vi "StateMachine_v01.vi"() -> ()   [LabVIEW 2014]
uses:
  StateMachine1Control.ctl
panel:
  out "ensaio":bool
  in  "waiting time":u32
  in  "currentCycleCtr":u32
  out "freio":bool
  in  "velocidade 2":u32
  out "velocidade":u32
  out "motor":bool
  in  "velocidade_inferior":u32
  in  "velocidade_superior":u32
  out "totalCycle":string
  out "currentCycle":string
  in  "numberOfCycles":u32 max=999 step=1 format="%0d"
  in  "stopButton":bool
  in  "startButton":bool
  out "state":T1
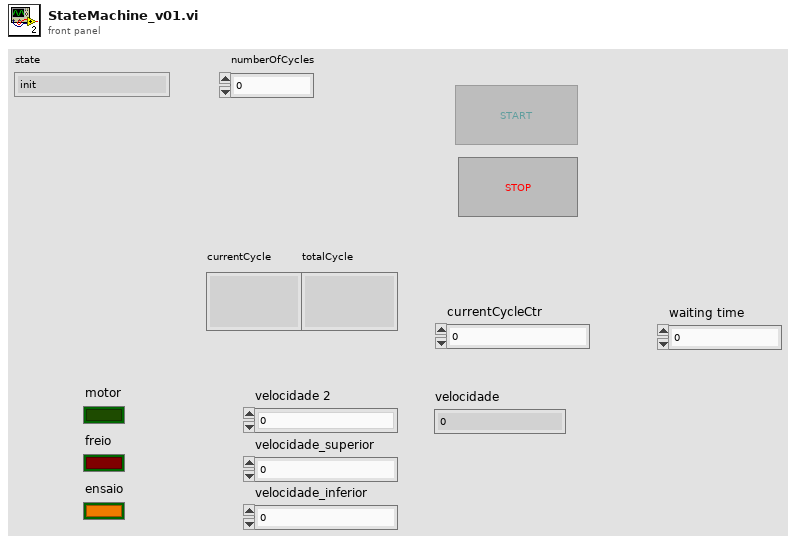
[diagram p1: front panel]
types:
  T1 = typedef "StateMachine1Control.ctl" = enum16{"init", "ready", "start motor cycle", "acquiring data", "start brake cycle", "finish", "shutdown"}
  T2 = enum8{"Enabled", "Disabled", "Disabled and Grayed Out"}
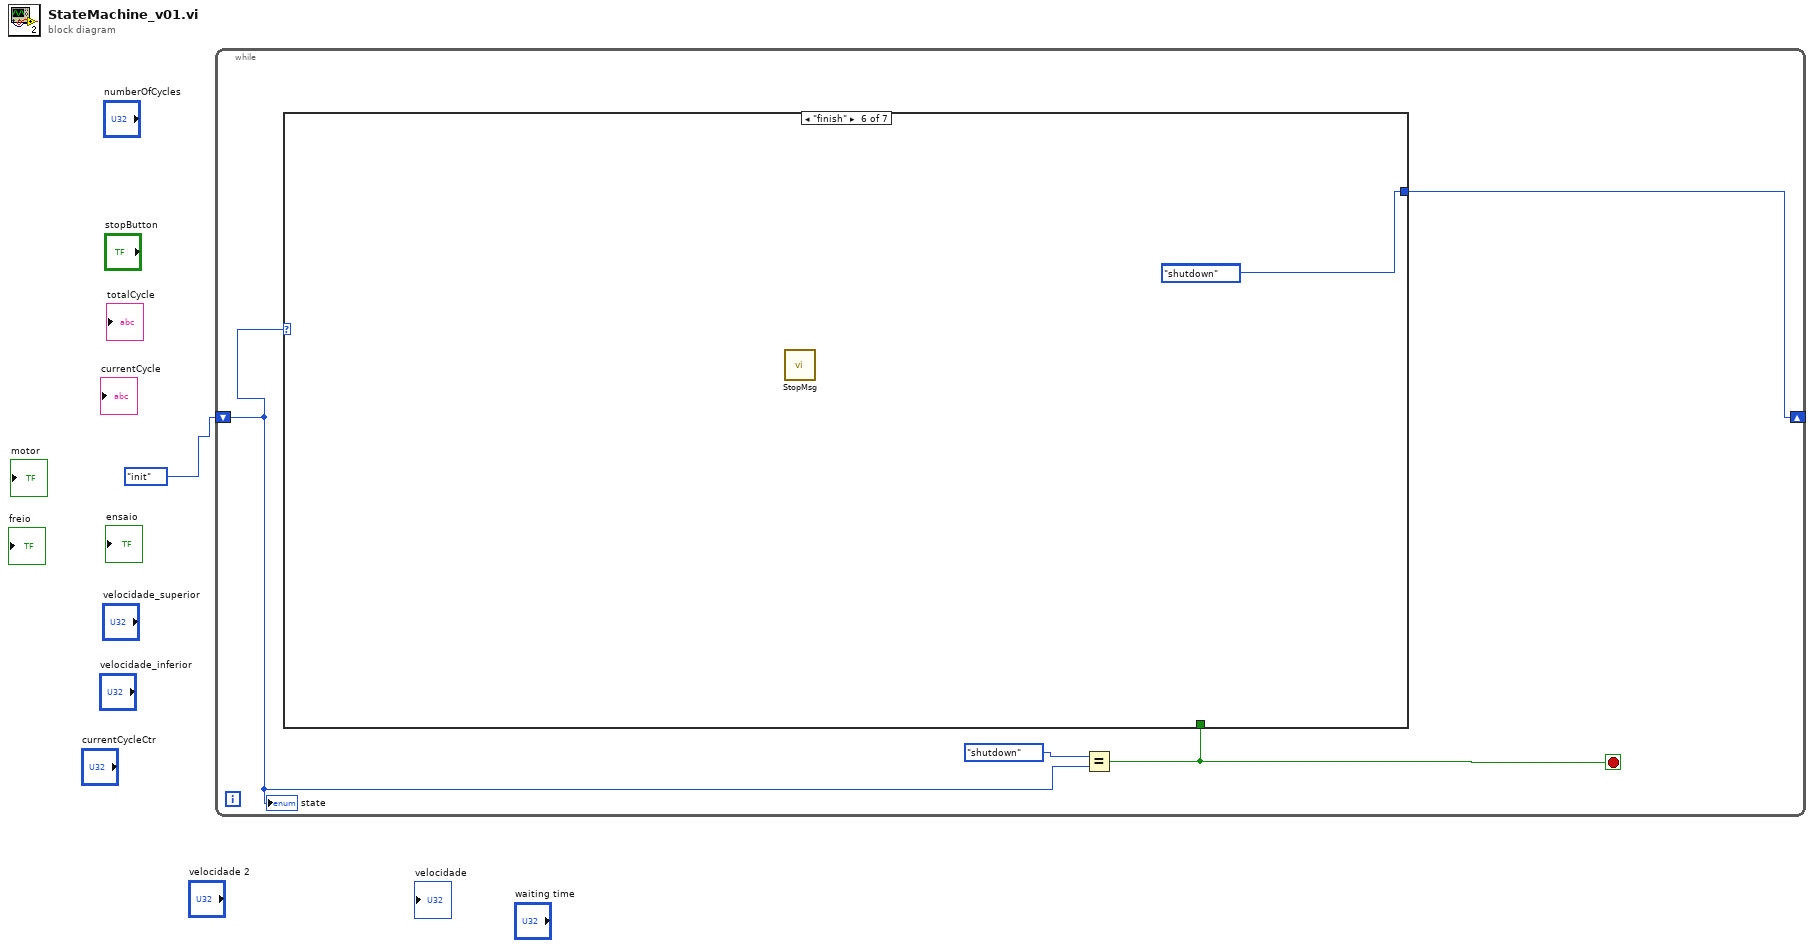
[diagram p0: block diagram]
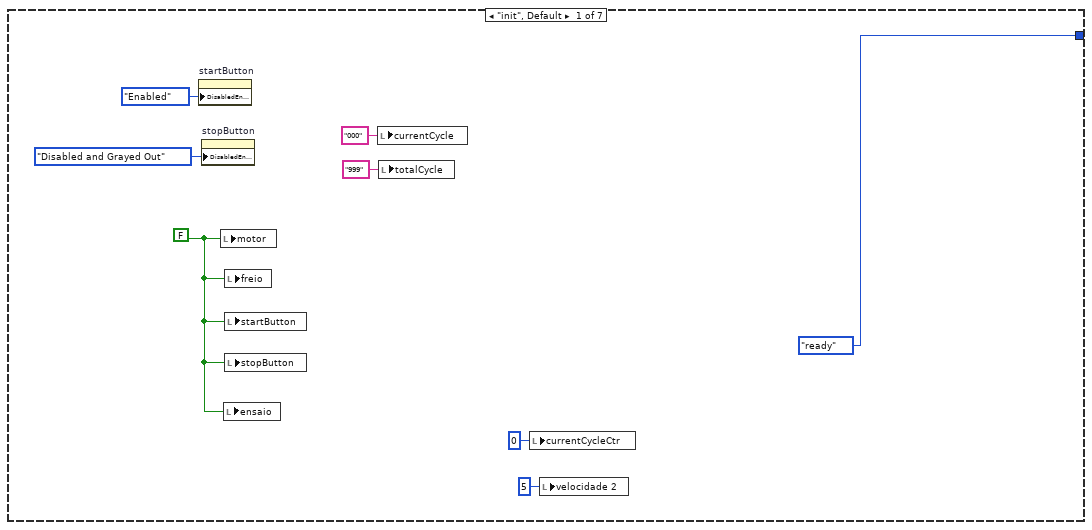
[diagram p2: hidden frame]
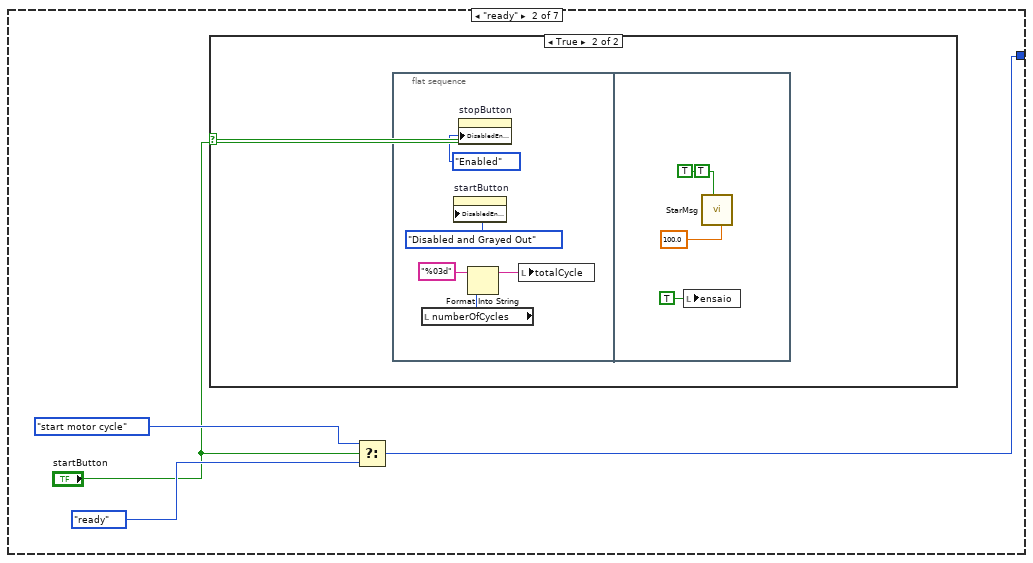
[diagram p3: hidden frame]
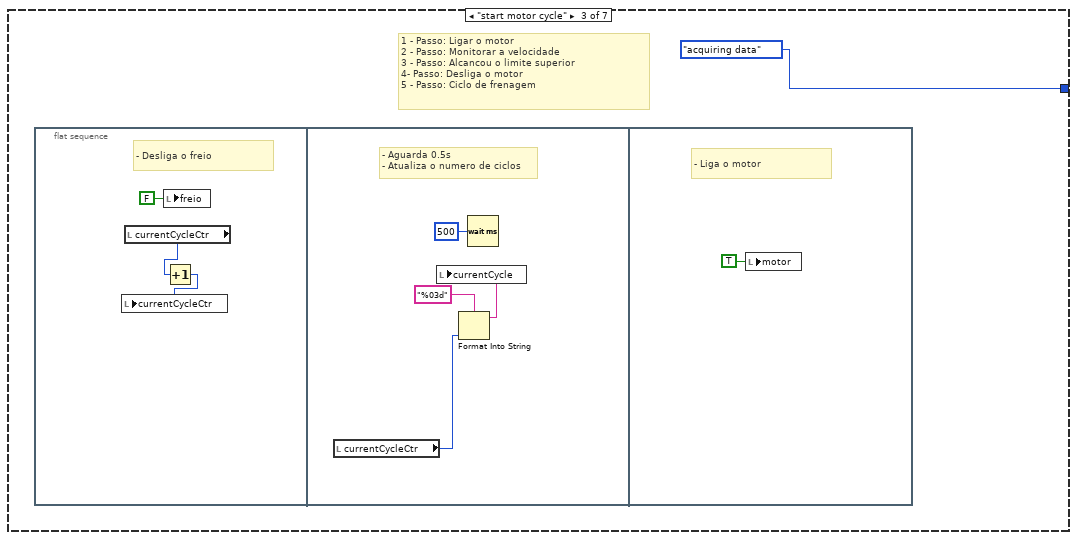
[diagram p5: hidden frame]
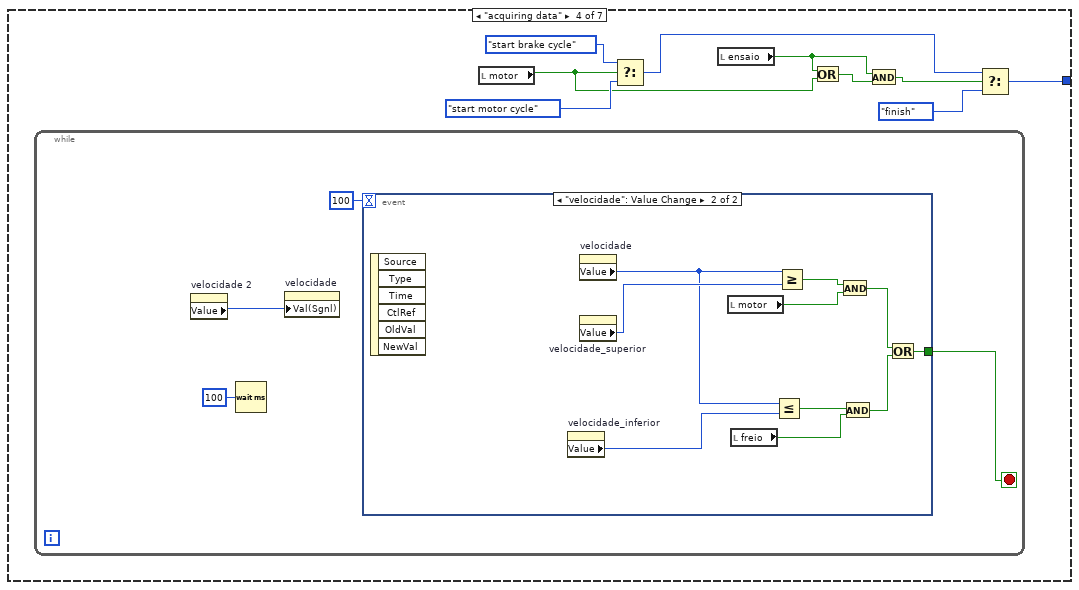
[diagram p6: hidden frame]
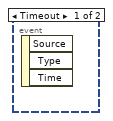
[diagram p7: hidden frame]
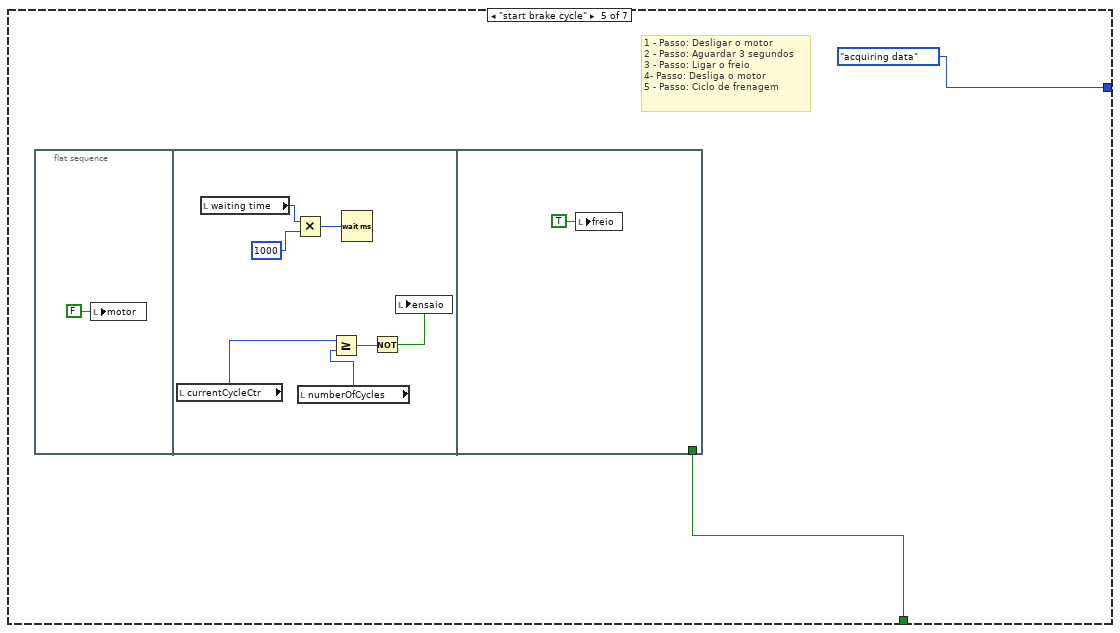
[diagram p8: hidden frame]
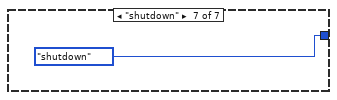
[diagram p9: hidden frame]
diagram:
  n1 = while {
    shift-right: [w2] -> _
    shift-left: StateMachine1Control."init" ("state") -> [w3]
    stop <- w4 stop-if-true
    n2 = Equal?(x=StateMachine1Control."shutdown" ("state"), y=w3) -> (x = y?=w4:bool)
    n3 = case shown="\"finish\"" w3 {
      tunnel: w4 -> [_ _ _ _ w59 _ _]
      tunnel: [StateMachine1Control."ready" ("state") w14 StateMachine1Control."acquiring data" ("state") w39 StateMachine1Control."acquiring data" ("state") StateMachine1Control."shutdown" ("state") StateMachine1Control."shutdown" ("state")] -> w2
      frame "init", Default {
        w7 = FALSE ("motor")
        n4 = property on="startButton" class="Bool (strict)"("DisabledEnum"=T2."Enabled" ("Disabled")) -> ()  [unwired: 2 in, 2 out]
        n5 = property on="stopButton" class="Bool (strict)"("DisabledEnum"=T2."Disabled and Grayed Out" ("Disabled")) -> ()  [unwired: 2 in, 2 out]
        n6 = local write "motor"(w7) -> ()
        n7 = local write "ensaio"(w7) -> ()
        n8 = local write "freio"(w7) -> ()
        n9 = local write "startButton"(w7) -> ()
        n10 = local write "stopButton"(w7) -> ()
        n11 = local write "currentCycle"("000" ("currentCycle")) -> ()
        n12 = local write "totalCycle"("999" ("totalCycle")) -> ()
        n13 = local write "currentCycleCtr"(u32 0 ("currentCycleCtr")) -> ()
        n14 = local write "velocidade 2"(u32 5 ("velocidade 2")) -> ()
      }
      frame "ready" {
        n15 = case shown="True" "startButton" {
          frame False {
          }
          frame True {
            n16 = flat-sequence {
              frame #0 {
                n17 = local read "numberOfCycles"() -> (w18:u32)
                n18 = property on="startButton" class="Bool (strict)"("DisabledEnum"=T2."Disabled and Grayed Out" ("Disabled")) -> ()  [unwired: 2 in, 2 out]
                n19 = property on="stopButton" class="Bool (strict)"("DisabledEnum"=T2."Enabled" ("Disabled")) -> ()  [unwired: 2 in, 2 out]
                n20 = Format Into String(format string="%03d", w18) -> (resulting string=w19:string)  [unwired: 2 in, 1 out]
                n21 = local write "totalCycle"(w19) -> ()
              }
              frame #1 {
                (unwired) TRUE ("Cancel Button (True)")
                n22 = local write "ensaio"(TRUE ("ensaio")) -> ()
                n23 = call "StarMsg.vi"("Show"=TRUE, "Max Value (100)"=100.0) -> ()  [unwired: 7 in, 2 out]
              }
            }
          }
        }
        n24 = Select(t=StateMachine1Control."start motor cycle" ("state"), s="startButton", f=StateMachine1Control."ready" ("state")) -> (s? t:f=w14:T1)
      }
      frame "start motor cycle" {
        # "1 - Passo: Ligar o motor\n2 - Passo: Monitorar a velocidade\n3 - Passo: Alcancou o limite superior\n4- Passo: Desliga o motor\n5 - Passo: Ciclo de frenagem"
        n25 = flat-sequence {
          frame #0 {
            # "- Desliga o freio"
            n26 = local read "currentCycleCtr"() -> (w28:u32)
            n27 = local write "freio"(FALSE ("freio")) -> ()
            n28 = Increment(x=w28) -> (x+1=w27:u32)
            n29 = local write "currentCycleCtr"(w27) -> ()
          }
          frame #1 {
            # "- Aguarda 0.5s \n- Atualiza o numero de ciclos"
            n30 = local read "currentCycleCtr"() -> (w30:u32)
            n31 = Format Into String(format string="%03d", w30) -> (resulting string=w31:string)  [unwired: 2 in, 1 out]
            n32 = local write "currentCycle"(w31) -> ()
            n33 = Wait (ms)(milliseconds to wait=u32 500) -> ()  [unwired: 1 out]
          }
          frame #2 {
            # "- Liga o motor"
            n34 = local write "motor"(TRUE ("motor")) -> ()
          }
        }
      }
      frame "acquiring data" {
        n35 = while {
          stop <- w44 stop-if-true
          n36 = property on="velocidade 2" class="DigNum (strict)"() -> ("Value"=w45:u32)  [unwired: 2 in, 2 out]
          n37 = Wait (ms)(milliseconds to wait=u32 100) -> ()  [unwired: 1 out]
          n38 = property on="velocidade" class="DigNum (strict)"("Val(Sgnl)"=w45) -> ()  [unwired: 2 in, 2 out]
          n39 = event shown="[1] \"velocidade\": Value Change" {
            selector: _ -> [_ _]
            dyn-events: _ -> [_ _]
            timeout: 100 -> [_ _]
            tunnel: [_ w48] -> w44
            event Timeout {
              n40 = event-data() -> ()  [unwired: 1 in, 3 out]
            }
            event "velocidade": Value Change {
              n41 = event-data() -> ()  [unwired: 1 in, 6 out]
              n42 = property on="velocidade_inferior" class="DigNum (strict)"() -> ("Value"=w53:u32)  [unwired: 2 in, 2 out]
              n43 = property on="velocidade" class="DigNum (strict)"() -> ("Value"=w54:u32)  [unwired: 2 in, 2 out]
              n44 = property on="velocidade_superior" class="DigNum (strict)"() -> ("Value"=w57:u32)  [unwired: 2 in, 2 out]
              n45 = local read "motor"() -> (w55:bool)
              n46 = local read "freio"() -> (w52:bool)
              n47 = Less Or Equal?(x=w54, y=w53) -> (x <= y?=w51:bool)
              n48 = Greater Or Equal?(x=w54, y=w57) -> (x >= y?=w56:bool)
              n49 = And(x=w56, y=w55) -> (x .and. y?=w49:bool)
              n50 = And(x=w51, y=w52) -> (x .and. y?=w50:bool)
              n51 = Or(x=w49, y=w50) -> (x .or. y?=w48:bool)
            }
          }
        }
        n52 = local read "motor"() -> (w38:bool)
        n53 = Select(t=StateMachine1Control."start brake cycle" ("state"), s=w38, f=StateMachine1Control."start motor cycle" ("state")) -> (s? t:f=w41:T1)
        n54 = local read "ensaio"() -> (w37:bool)
        n55 = Or(x=w37, y=w38) -> (x .or. y?=w36:bool)
        n56 = And(x=w37, y=w36) -> (x .and. y?=w35:bool)
        n57 = Select(t=w41, s=w35, f=StateMachine1Control."finish" ("state")) -> (s? t:f=w39:T1)
      }
      frame "start brake cycle" {
        # "1 - Passo: Desligar o motor\n2 - Passo: Aguardar 3 segundos\n3 - Passo: Ligar o freio\n4- Passo: Desliga o motor\n5 - Passo: Ciclo de frenagem"
        n58 = flat-sequence {
          tunnel: w59 -> [_]
          frame #0 {
            n59 = local write "motor"(FALSE ("motor")) -> ()
          }
          frame #1 {
            n60 = local read "currentCycleCtr"() -> (w64:u32)
            n61 = local read "waiting time"() -> (w67:u32)
            n62 = Multiply(x=w67, y=u32 1000) -> (x*y=w65:u32)
            n63 = local read "numberOfCycles"() -> (w63:u32)
            n64 = Greater Or Equal?(x=w64, y=w63) -> (x >= y?=w62:bool)
            n65 = Wait (ms)(milliseconds to wait=w65) -> ()  [unwired: 1 out]
            n66 = Not(x=w62) -> (.not. x?=w61:bool)
            n67 = local write "ensaio"(w61) -> ()
          }
          frame #2 {
            n68 = local write "freio"(TRUE ("freio")) -> ()
          }
        }
      }
      frame "finish" {
        (unwired) StateMachine1Control."shutdown" ("state")
        n69 = call "StopMsg.vi"() -> ()  [unwired: 9 in, 2 out]
      }
      frame "shutdown" {
      }
    }
    "state" <- w3
  }
